vi "ORS_set_file_position.vi"(8 "current B-scan":i32=1, 9 "file version":u32=2, 11 "Cluster":T1) -> (0 "B-data skip":dbl, 3 "refnum out":refnum<file>)   [LabVIEW 2014]
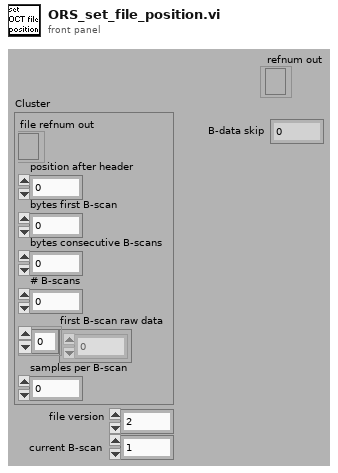
[diagram p1: front panel]
types:
  T1 = cluster{"file refnum out":refnum<file>, "position after header":i64, "bytes first B-scan":i64, "bytes consecutive B-scans":i64, "# B-scans":i32, "first B-scan raw data":i16[], "samples per B-scan":i32}
  T2 = enum16{"big-endian, network order", "native, host order", "little-endian"}
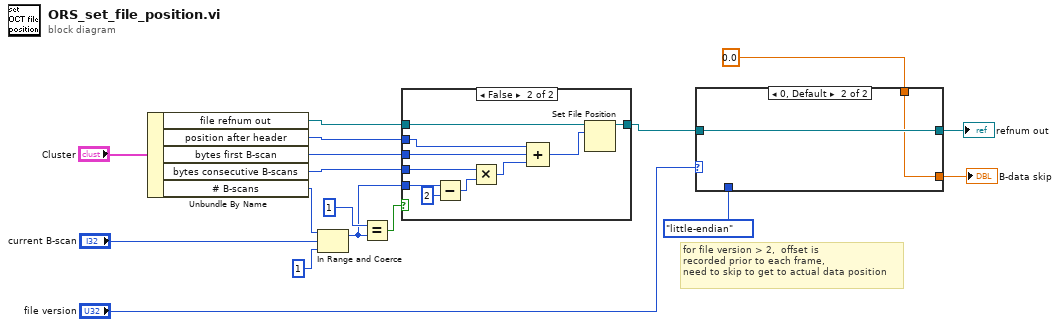
[diagram p0: block diagram]
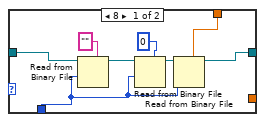
[diagram p2: hidden frame]
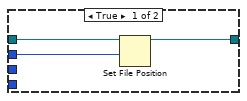
[diagram p3: hidden frame]
diagram:
  # "for file version > 2,  offset is \nrecorded prior to each frame,\nneed to skip to get to actual data position"
  n1 = Unbundle By Name("Cluster") -> ("file refnum out"=w11:refnum<file>, "position after header"=w10:i64, "bytes first B-scan"=w9:i64, "bytes consecutive B-scans"=w7:i64, "# B-scans"=w16:i32)
  n2 = In Range and Coerce(upper limit=w16, x="current B-scan", lower limit=1) -> (coerced(x)=w8:i32)  [unwired: 1 out]
  n3 = Equal?(x=1, y=w8) -> (x = y?=w12:bool)
  n4 = case shown="False" w12 {
    tunnel: w11 -> [w20 w30]
    tunnel: w10 -> [w19 w25]
    tunnel: w9 -> [_ w24]
    tunnel: w8 -> [_ w29]
    tunnel: w7 -> [_ w27]
    tunnel: [w18 w21] -> w4
    frame True {
      n5 = Set File Position(offset (in bytes) (0)=w19, refnum=w20) -> (refnum out=w18:refnum<file>)  [unwired: 2 in, 1 out]
    }
    frame False {
      n6 = Subtract(x=w29, y=2) -> (x-y=w26:i32)
      n7 = Multiply(x=w27, y=w26) -> (x*y=w23:i64)
      n8 = Compound Arithmetic op=ADD(w25, w24, w23) -> (w22:i64)
      n9 = Set File Position(offset (in bytes) (0)=w22, refnum=w30) -> (refnum out=w21:refnum<file>)  [unwired: 2 in, 1 out]
    }
  }
  n10 = case shown="0, Default" "file version" {
    tunnel: [w35 w40] -> w1
    tunnel: T2."little-endian" ("byte order (0:big-endian, network order)") -> [w31 _]
    tunnel: w4 -> [w38 w40]
    tunnel: 0.0 -> [w33 w39]
    tunnel: [_ w39] -> w2
    frame 8 {
      n11 = Read from Binary File(5:"", 9:w31, 11:w38) -> (3:w37:refnum<file>)  [unwired: 3 in, 3 out]
      n12 = Read from Binary File(5:u64 0, 9:w31, 11:w37) -> (3:w36:refnum<file>)  [unwired: 3 in, 3 out]
      n13 = Read from Binary File(5:w33, 9:w31, 11:w36) -> (3:w35:refnum<file>)  [unwired: 3 in, 3 out]
    }
    frame 0, Default {
    }
  }
  "refnum out" <- w1
  "B-data skip" <- w2
